vi "RSZVB Write Limit Line Segment List.vi"(0 "VISA session":refnum<visa-resource-name>, 1 "Stop Stimulus":dbl[](array[numeric]) format="%^.3e", 2 "Stop Response":dbl[](array[numeric]) format="%^.3e", 5 "Channel (Trace) (1)":i32=1, 9 "Type (1: Upper)":i32(ring)=1 items=["Upper"=1, "Lower"=2], 11 "error in (no error)":errorcluster {"code" format="%.0x"}, 12 "Start Response":dbl[](array[numeric]) format="%^.3e", 13 "Start Stimulus":dbl[](array[numeric]) format="%^.3e") -> (4 "dup VISA session":refnum<visa-resource-name>, 15 "error out":errorcluster {"code" format="%.0x"})   [LabVIEW 2011]
doc: "This VI defines the stimulus values of the limit line and/or creates new limit line segments. It also defines the response (y-axis) values of the lower (upper) limit line.\n\nNote(s):\n\n(1) This VI use a fixed numbering scheme for limit line segments: Upper limit line segments are assigned odd numbers (1, 3, 5,...), lower limit line segments are assigned even numbers (2, 4, 6,...).\n\n(2) Rules for creating segments:\nThe following rules apply to an active trace with n existing upper and n existing lower limit line segments:\n\nAn odd number of values is rejected; an error message -109,\"Missing parameter...\" is generated. \n\nAn even number of 2*k values updates or generates k lower limit line segments. \n\nFor n > k the response values of all existing lower limit line segments no. 2, 4, ...,2*k are updated, the existing upper and lower limit line segments no. 2*k+1, ..., 2*n are deleted. The existing upper limit line segments no. 1, 3, 2*k-1 are not affected. \n\nFor n < k the response values of the lower limit line segments no. 2, 4 to 2*n are updated, the lower limit line segments 2*n+2, 2*n+4,..., 2*k are generated with default stimulus values (see CALCulate<Ch/Tr>:LIMit:CONTrol[:DATA] . In addition, the missing upper limit line segments 2*n+1, 2*n+3,..., 2*k-1 are generated with default stimulus and response values \n\nRemote-control command(s):\nCALCulate<Ch/Tr>:LIMit:CONTrol[:DATA] <numeric_value>,<numeric_value>{,<numeric_value>,<numeric_value>}\nCALCulate<Ch/Tr>:LIMit:LOWer[:DATA] <numeric_value>,<numeric_value>{,<numeric_value>,<numeric_value>}\nCALCulate<Ch/Tr>:LIMit:UPPer[:DATA] <numeric_value>,<numeric_value>{,<numeric_value>,<numeric_value>}"
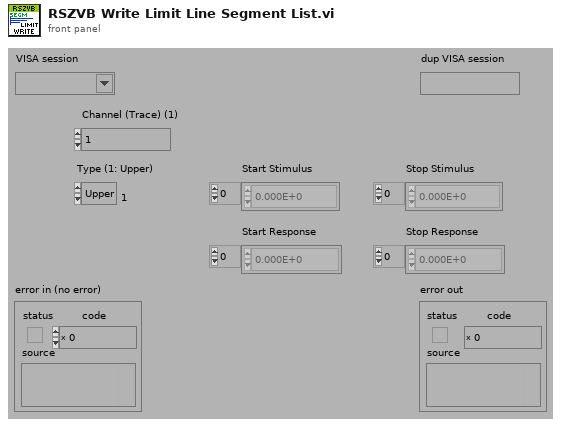
[diagram p1: front panel]
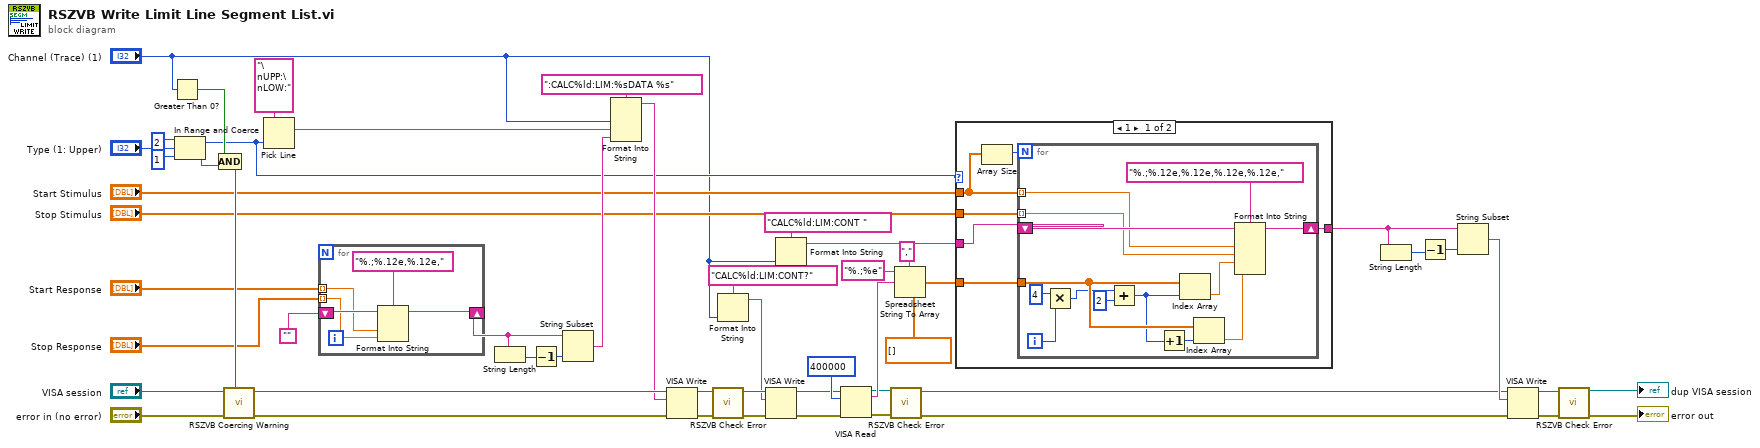
[diagram p0: block diagram]
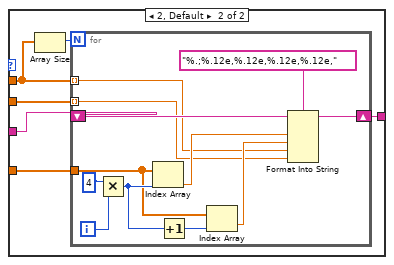
[diagram p2: hidden frame]
diagram:
  n1 = Greater Than 0?(x="Channel (Trace) (1)") -> (x > 0?=w43:bool)
  n2 = In Range and Coerce(upper limit=2, x="Type (1: Upper)", lower limit=1) -> (coerced(x)=w20:i32, In Range?=w46:bool)
  n3 = Compound Arithmetic op=AND(w43, w46) -> (w45:bool)
  n4 = call "RSZVB Coercing Warning.vi"("In Range?"=w45, "error in (no error)"="error in (no error)", "VISA session"="VISA session") -> ("error out"=w52:errorcluster, "dup VISA session"=w53:refnum<visa-resource-name>)  [unwired: 7 in]
  n5 = Pick Line(multi-line string="\nUPP:\nLOW:", line index=w20) -> (output string=w32:string)  [unwired: 1 in]
  n6 = for {
    tunnel: "Start Response" -> [w54] mode=indexing
    tunnel: "Stop Response" -> [w55] mode=indexing
    shift-right: [w57] -> w34
    shift-left: "" -> [w56]
    n7 = Format Into String(format string="%.;%.12e,%.12e,", initial string=w56, w54, w55) -> (resulting string=w57:string)  [unwired: 1 in, 1 out]
  }
  n8 = String Length(string=w34) -> (length=w36:i32)
  n9 = Decrement(x=w36) -> (x-1=w35:i32)
  n10 = String Subset(string=w34, length (rest)=w35) -> (substring=w31:string)  [unwired: 1 in]
  n11 = Format Into String(format string=":CALC%ld:LIM:%sDATA %s", "Channel (Trace) (1)", w32, w31) -> (resulting string=w44:string)  [unwired: 2 in, 1 out]
  n12 = VISA Write(VISA resource name=w53, write buffer=w44, error in (no error)=w52) -> (VISA resource name out=w50:refnum<visa-resource-name>, error out=w51:errorcluster)  [unwired: 1 out]
  n13 = call "RSZVB Check Error.vi"("error in (no error)"=w51, "VISA session"=w50) -> ("error out"=w27:errorcluster, "dup VISA session"=w26:refnum<visa-resource-name>)  [unwired: 8 in]
  n14 = Format Into String(format string="CALC%ld:LIM:CONT?" ("write buffer (\"\")"), "Channel (Trace) (1)") -> (resulting string=w24:string)  [unwired: 2 in, 1 out]
  n15 = VISA Write(VISA resource name=w26, write buffer=w24, error in (no error)=w27) -> (VISA resource name out=w1:refnum<visa-resource-name>, error out=w23:errorcluster)  [unwired: 1 out]
  n16 = Format Into String(format string="CALC%ld:LIM:CONT " ("write buffer (\"\")"), "Channel (Trace) (1)") -> (resulting string=w15:string)  [unwired: 2 in, 1 out]
  n17 = VISA Read(VISA resource name=w1, byte count=u32 400000 ("byte count (0)"), error in (no error)=w23) -> (VISA resource name out=w10:refnum<visa-resource-name>, read buffer=w29:string, error out=w9:errorcluster)  [unwired: 1 out]
  n18 = call "RSZVB Check Error.vi"("error in (no error)"=w9, "VISA session"=w10) -> ("error out"=w7:errorcluster, "dup VISA session"=w8:refnum<visa-resource-name>)  [unwired: 8 in]
  n19 = Spreadsheet String To Array(delimiter (Tab)=",", format string="%.;%e", spreadsheet string=w29, array type (2D Dbl)=dbl[] []) -> (array=w21:dbl[])
  n20 = case shown="1" w20 {
    tunnel: w21 -> [w64 w84]
    tunnel: "Start Stimulus" -> [w61 w81]
    tunnel: "Stop Stimulus" -> [w63 w83]
    tunnel: w15 -> [w60 w80]
    tunnel: [w59 w79] -> w12
    frame 1 {
      n21 = Array Size(array=w61) -> (size(s)=w62:i32)
      n22 = for {
        N: w62 -> [_]
        tunnel: w64 -> [w68]
        tunnel: w61 -> [w75] mode=indexing
        tunnel: w63 -> [w74] mode=indexing
        shift-right: [w76] -> w59
        shift-left: w60 -> [w77]
        i -> [w71]
        n23 = Multiply(x=4 ("y"), y=w71) -> (x*y=w67:i32)
        n24 = Add(x=w67, y=2) -> (x+y=w65:i32)
        n25 = Increment(x=w65) -> (x+1=w72:i32)
        n26 = Index Array(array=w68, index=w65) -> (element=w73:dbl)
        n27 = Index Array(array=w68, index=w72) -> (element=w69:dbl)
        n28 = Format Into String(format string="%.;%.12e,%.12e,%.12e,%.12e,", initial string=w77, w75, w74, w73, w69) -> (resulting string=w76:string)  [unwired: 1 in, 1 out]
      }
    }
    frame 2, Default {
      n29 = Array Size(array=w81) -> (size(s)=w82:i32)
      n30 = for {
        N: w82 -> [_]
        tunnel: w84 -> [w89]
        tunnel: w81 -> [w86] mode=indexing
        tunnel: w83 -> [w85] mode=indexing
        shift-right: [w94] -> w79
        shift-left: w80 -> [w95]
        i -> [w91]
        n31 = Multiply(x=4 ("y"), y=w91) -> (x*y=w93:i32)
        n32 = Index Array(array=w89, index=w93) -> (element=w88:dbl)
        n33 = Increment(x=w93) -> (x+1=w92:i32)
        n34 = Index Array(array=w89, index=w92) -> (element=w87:dbl)
        n35 = Format Into String(format string="%.;%.12e,%.12e,%.12e,%.12e,", initial string=w95, w88, w87, w86, w85) -> (resulting string=w94:string)  [unwired: 1 in, 1 out]
      }
    }
  }
  n36 = String Length(string=w12) -> (length=w13:i32)
  n37 = Decrement(x=w13) -> (x-1=w14:i32)
  n38 = String Subset(string=w12, length (rest)=w14) -> (substring=w11:string)  [unwired: 1 in]
  n39 = VISA Write(VISA resource name=w8, write buffer=w11, error in (no error)=w7) -> (VISA resource name out=w6:refnum<visa-resource-name>, error out=w5:errorcluster)  [unwired: 1 out]
  n40 = call "RSZVB Check Error.vi"("error in (no error)"=w5, "VISA session"=w6) -> ("error out"=→"error out":errorcluster, "dup VISA session"=→"dup VISA session":refnum<visa-resource-name>)  [unwired: 8 in]
